vi "Auto Clear SMU Trigger Model Event Detector.vi"(8 "error in (no error)":errorcluster, 9 "Auto Clear Detector (F: Disable)":bool, 10 "Source Measure Unit Channel (0: Channel A)":i32(ring) items=["Channel A", "Channel B"], 11 "VISA resource name":refnum<visa-resource-name>) -> (0 "error out":errorcluster, 3 "VISA resource name out":refnum<visa-resource-name>)   [LabVIEW 2015, in "Keithley 2600 Series.lvlib"]
doc: "Turns automatic clearing of the event detectors on or off."
uses:
  Keithley 2600 Series.lvlib
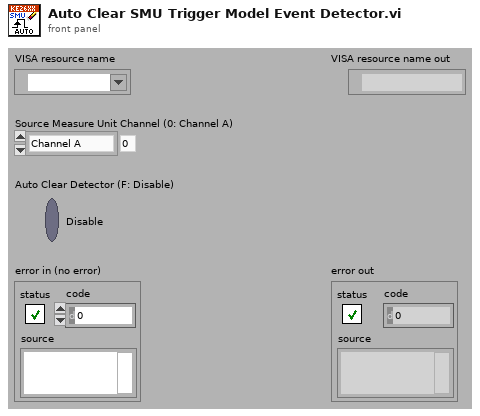
[diagram p1: front panel]
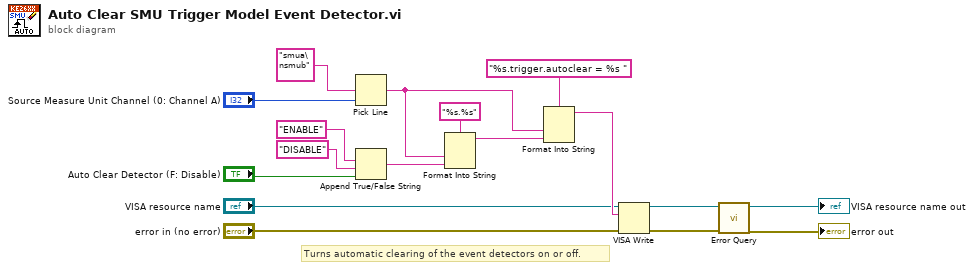
[diagram p0: block diagram]
diagram:
  # "Turns automatic clearing of the event detectors on or off."
  n1 = Pick Line(multi-line string="smua\nsmub", line index="Source Measure Unit Channel (0: Channel A)") -> (output string=w2:string)  [unwired: 1 in]
  n2 = Append True/False String(1:"Auto Clear Detector (F: Disable)", 2:"DISABLE", 3:"ENABLE") -> (0:w3:string)  [unwired: 1 in]
  n3 = Format Into String(format string="%s.%s", w2, w3) -> (resulting string=w1:string)  [unwired: 2 in, 1 out]
  n4 = Format Into String(format string="%s.trigger.autoclear = %s ", w2, w1) -> (resulting string=w13:string)  [unwired: 2 in, 1 out]
  n5 = VISA Write(VISA resource name="VISA resource name", write buffer=w13, error in (no error)="error in (no error)") -> (VISA resource name out=w10:refnum<visa-resource-name>, error out=w9:errorcluster)  [unwired: 1 out]
  n6 = call "Error Query.vi"("error in (no error)"=w9, "VISA resource name"=w10) -> ("error out"=→"error out":errorcluster, "VISA resource name out"=→"VISA resource name out":refnum<visa-resource-name>)  [unwired: 6 in, 2 out]
